vi "Theme5_Topic1_qn9.vi"(9 "RefPrevious":refnum<vi>, 10 "RefNext":refnum<vi>, 11 "connection reference":T1) -> (2 "AnsIndicator":refnum<vi>[](array[refnum]))   [LabVIEW 2013]
uses:
  Precontrol.vi
  <vilib>/addons/database/Connection.llb/Conn ObjectReference.ctl
  <vilib>/addons/database/NI_Database_API.lvlib
panel:
  out "Header":string[][](table)
  out "MCQ_RandomizedTbl":string[][](table)
  out "DInd":bool
  out "CInd":bool
  out "BInd":bool
  out "AInd":bool
  in  "ABCD":enum32{"No Selection", "A", "B", "C", "D"}(radio)
  # "Two table-tennis balls, R and S, are coated with aluminium paint ane are suspended by\nnylon threads. Each ball is given a charge and the balls come to rest in the position as\nshown in the diagram below."
  # "Which of the following correctly shows the sign and quntity of the charge on balls R and \nS respectively?"
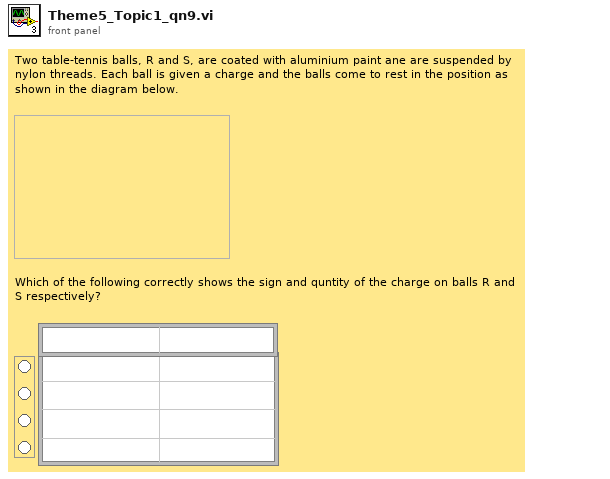
[diagram p1: front panel]
types:
  T1 = typedef "NI_Database_API.lvlib/Conn ObjectReference.ctl" = refnum<k1>
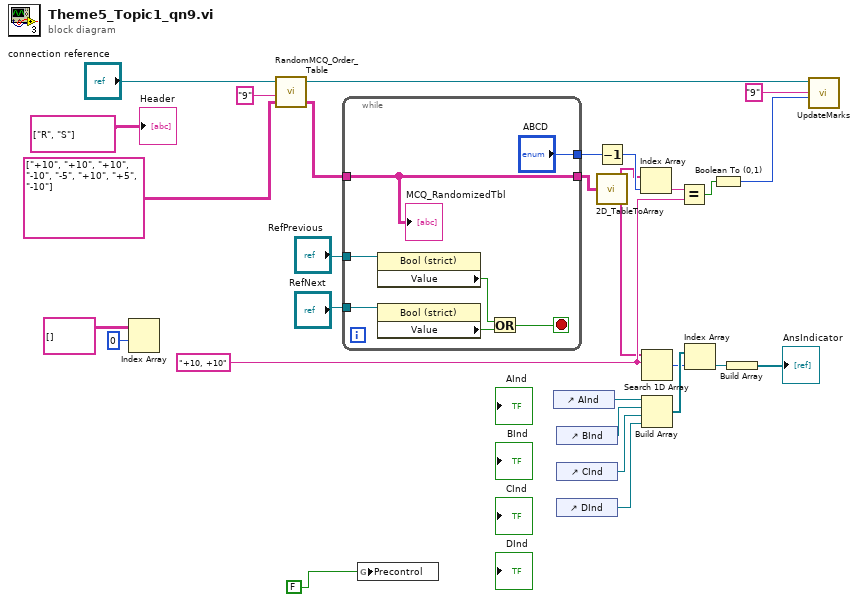
[diagram p0: block diagram]
diagram:
  w7 = "+10, +10" ("element")
  n1 = Index Array(array=string[][] [], index (row)=0) -> ()  [unwired: 1 in, 1 out]
  n2 = call "RandomMCQ_Order_Table.vi"("MCQ_Ordered"=string[][] [["+10", "+10"], ["+10", "-10"], ["-5", "+10"], ["+5", "-10"]] ("MCQ_Randomized"), "Questions_Ordered"="9", "connection reference"="connection reference") -> ("MCQ_Randomized"=w28:string[][], "connection reference out"=w14:T1)  [unwired: 1 in]
  n3 = while {
    tunnel: ["ABCD"] -> w18
    tunnel: w28 -> [w29]
    tunnel: [w29] -> w8
    tunnel: "RefNext" -> [w31]
    tunnel: "RefPrevious" -> [w32]
    stop <- w30 stop-if-true
    n4 = property class="Bool (strict)"(reference=w32) -> ("Value"=w34:bool)  [unwired: 1 in, 2 out]
    n5 = property class="Bool (strict)"(reference=w31) -> ("Value"=w33:bool)  [unwired: 1 in, 2 out]
    n6 = Or(x=w34, y=w33) -> (x .or. y?=w30:bool)
    "MCQ_RandomizedTbl" <- w29
  }
  n7 = global write "Precontrol.vi" "Precontrol"(FALSE) -> ()
  n8 = control-ref of="AInd"() -> (w25:refnum<vi>)
  n9 = control-ref of="BInd"() -> (w24:refnum<vi>)
  n10 = control-ref of="CInd"() -> (w23:refnum<vi>)
  n11 = control-ref of="DInd"() -> (w22:refnum<vi>)
  n12 = Decrement(x=w18) -> (x-1=w11:enum32{"No Selection", "A", "B", "C", "D"})
  n13 = call "2D_TableToArray.vi"("TableIn"=w8) -> ("\"col1\", \"col2\""=w6:string[])
  n14 = Index Array(array=w6, index=w11) -> (element=w17:string)
  n15 = Search 1D Array(1D array=w6, element=w7) -> (index of element=w20:i32)  [unwired: 1 in]
  n16 = Build Array(w25, w24, w23, w22) -> (w21:refnum<vi>[])
  n17 = Equal?(x=w17, y=w7) -> (x = y?=w3:bool)
  n18 = Index Array(array=w21, index=w20) -> (element=w19:refnum<vi>)
  n19 = Boolean To (0,1)(Boolean=w3) -> (0, 1=w2:i16)
  n20 = Build Array(w19) -> (→"AnsIndicator":refnum<vi>[])
  n21 = call "UpdateMarks.vi"("MarksEarned"=w2, "QuestionsNo_Ordered"="9", "connection reference"=w14) -> ()  [unwired: 9 in]
  "Header" <- string[][] [["R", "S"]] ("MCQ_Randomized")
